vi "datasource.create.vi"(8 "error in":errorcluster, 9 "Description":string, 10 "ID":string, 11 "Nominal Client in":refnum<class "Nominal Client.lvclass">) -> (0 "error out":errorcluster, 1 "Response":string, 2 "Response Headers":refnum<class "Response Headers.lvclass">, 3 "Nominal Client out":refnum<class "Nominal Client.lvclass">)   [LabVIEW 2020, in "Nominal Client.lvclass"]
uses:
  Nominal Client.lvclass
  <vilib>/addons/_JKI.lib/REST Client/classes/Response Headers/Response Headers.lvclass
  Nominal Client.lvclass/Nominal Client.ctl
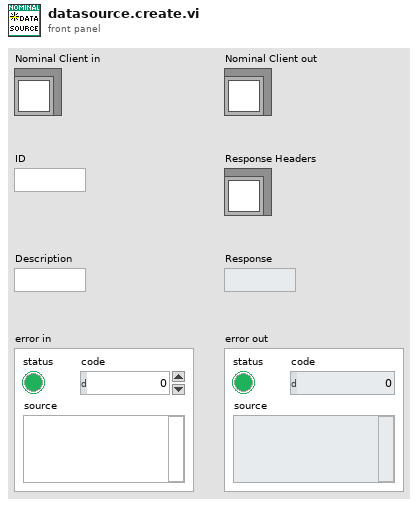
[diagram p1: front panel]
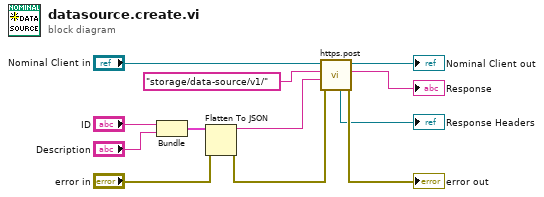
[diagram p0: block diagram]
diagram:
  n1 = Bundle("ID"="ID", "Description"="Description") -> (w7:cluster{"ID":string, "Description":string})  [unwired: 1 in]
  n2 = Flatten To JSON(anything=w7, error in (no error)="error in") -> (JSON string=w8:string, 11:w1:errorcluster)  [unwired: 1 in]
  n3 = call "https.post.vi"("error in"=w1, "Request body"=w8, "Path"="storage/data-source/v1/", "Nominal Client in"="Nominal Client in") -> ("error out"=→"error out":errorcluster, "Response"=→"Response":string, "Nominal Client out"=→"Nominal Client out":refnum<class "Nominal Client.lvclass">, "Response Headers"=→"Response Headers":refnum<class "Response Headers.lvclass">)  [unwired: 4 in]
